vi "34970 Error Query++.vi"(0 "VISA session":refnum<visa-resource-name>, 11 "error in (no error)":errorcluster) -> (4 "dup VISA session":refnum<visa-resource-name>, 8 "Error":i32, 10 "Error Message":string, 15 "error out":errorcluster)   [LabVIEW 2020]
doc: "This VI reads an error from the instrument. It expects to see errors in SCPI format (#,\"error message\"). If an error query is not supported, it returns a warning.\n\nModified to silence output to error cluster if no error present.\nW. Gilbert, University of Minnesota Physics, 8/6/2004\nwgilbert@physics.umn.edu"
panel:
  out "read buffer":string
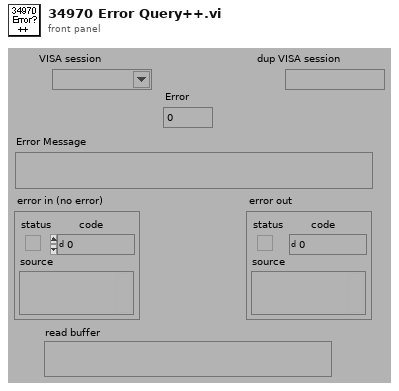
[diagram p1: front panel]
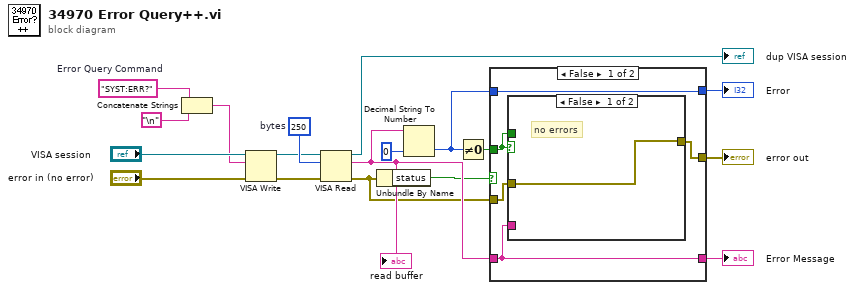
[diagram p0: block diagram]
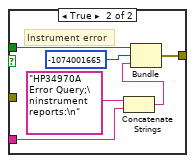
[diagram p2: hidden frame]
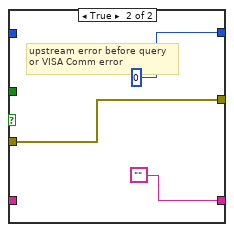
[diagram p3: hidden frame]
diagram:
  w7 = u32 250  # bytes
  w3 = "SYST:ERR?"  # Error Query Command
  n1 = Concatenate Strings(w3, "\n") -> (w1:string)
  n2 = VISA Write(VISA resource name="VISA session", write buffer=w1, error in (no error)="error in (no error)") -> (VISA resource name out=w6:refnum<visa-resource-name>, error out=w8:errorcluster)  [unwired: 1 out]
  n3 = VISA Read(VISA resource name=w6, byte count=w7, error in (no error)=w8) -> (VISA resource name out=→"dup VISA session":refnum<visa-resource-name>, read buffer=w11:string, error out=w5:errorcluster)  [unwired: 1 out]
  "read buffer" <- w11
  n4 = Unbundle By Name(w5) -> ("status"=w9:bool)
  n5 = Decimal String To Number(string=w11, default (0L)=0) -> (number=w4:i32)  [unwired: 2 out]
  n6 = Not Equal To 0?(x=w4) -> (x != 0?=w10:bool)
  n7 = case shown="False" w9 {
    tunnel: w11 -> [w19 _]
    tunnel: w5 -> [w20 w33]
    tunnel: [w23 w33] -> w13
    tunnel: [w19 ""] -> w18
    tunnel: [w22 0] -> w17
    tunnel: w4 -> [w22 _]
    tunnel: w10 -> [w21 _]
    frame False {
      n8 = case shown="False" w21 {
        tunnel: w19 -> [_ w25]
        tunnel: [w24 w27] -> w23
        tunnel: w21 -> [_ w26]
        tunnel: w20 -> [w24 _]
        frame False {
          # "no errors"
        }
        frame True {
          # "Instrument error"
          n9 = Concatenate Strings("HP34970A Error Query;\ninstrument reports:\n", w25) -> (w28:string)
          n10 = Bundle(w26, -1074001665, w28) -> (w27:errorcluster)  [unwired: 1 out]
        }
      }
    }
    frame True {
      # "upstream error before query\nor VISA Comm error"
    }
  }
  "Error Message" <- w18
  "Error" <- w17
  "error out" <- w13
